vi "PathPlanner_PathFinder_DefaultFieldSize.vi"() -> (1 "fieldWidth_Meters":dbl, 3 "fieldLength_Meters":dbl)   [LabVIEW 2019, in "PathPlanner24.lvlib"]
doc: "Internal function. Not to be used by end users."
uses:
  PathPlanner24.lvlib
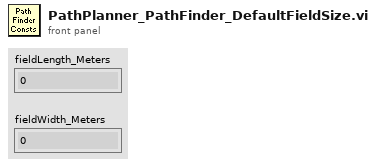
[diagram p1: front panel]
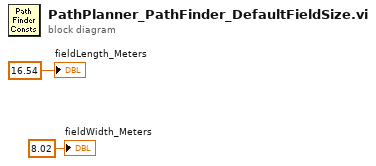
[diagram p0: block diagram]
diagram:
  "fieldLength_Meters" <- 16.54 ("SMOOTHING_ANCHOR_PCT")
  "fieldWidth_Meters" <- 8.02 ("SMOOTHING_CONTROL_PCT")
